vi "_old_Load_SetList_SubVI_Getv2_v4.vi"(0 "Path":path, 1 "error in (no error)":errorcluster) -> (2 "Procedure Name":string="IBS_PICameraTest_29Sep04", 3 "Paramaters":T1 {"Agilent built-in fxns array"."Ring" items=["Agilent", "Rohde & Schwarz"]; "Agilent built-in fxns array"."Agilent phase shift parameter"."FSK pulse length [s]" min=1e-06 max=80000000.0 format="%.3p"; "Agilent built-in fxns array"."Agilent phase shift parameter"."Phase [deg]" min=1e-06 max=80000000.0 format="%.3p"; "Agilent built-in fxns array"."Function selection" items=["Fixed waveform", "Frequency sweep", "Phase shift"]; "Agilent built-in fxns array"."Agilent selection" items=["Raman"]; "Agilent built-in fxns array"."Agilent fixed waveform parameters"."Amplitude [Vpp]" min=0.001 max=20.0 format="%.2f"; "Agilent built-in fxns array"."Agilent fixed waveform parameters"."Waveform Shape" items=["DC"=0, "Sine"=1, "Square"=2, "Triangle"=3, "Ramp"=4, "Pulse"=6, "Noise"=7, "Sinc"=8, "Neg. Ramp"=9, "Exp. Rise"=10, "Exp. Fall"=11, "Cardiac"=12, "Volatile"=13, "User Def. Wfm"=14]; "Agilent built-in fxns array"."Agilent fixed waveform parameters"."Offset [V]" min=-10.0 max=10.0 format="%.2f"; "Agilent built-in fxns array"."Agilent fixed waveform parameters"."Frequency [Hz]" min=0.0001 max=80000000.0 format="%.6p"; "Agilent built-in fxns array"."Agilent sweep parameters"."Sweep Time [s]" min=0.001 max=500.0 format="%.3p"; "Agilent built-in fxns array"."Agilent sweep parameters"."Sweep Spacing (0: Linear up)" items=["Linear up", "Log up", "Linear down", "Log down"]; "Agilent built-in fxns array"."Agilent sweep parameters"."Sweep Mode (0: Off)" items=["Off", "Int", "Ext", "Bus"]; "Agilent built-in fxns array"."Agilent sweep parameters"."Upper Frequency [Hz][1]" min=1e-06 max=80000000.0 format="%.6p"; "Agilent built-in fxns array"."Agilent sweep parameters"."Lower Frequency [Hz][0]" min=1e-06 max=80000000.0 format="%.6p"; "SRS Ramps"."lattice ramp"."c" format="%.2p"; "SRS Ramps"."lattice ramp"."b" format="%.2p"; "SRS Ramps"."lattice ramp"."dt" format="%.2p"; "SRS Ramps"."lattice ramp"."a" format="%.2p"; "Sequencing Info"."Computed Step Size" format="%.2p"; "Sequencing Info"."Sequenced Data" format="%.2p"; "Sequencing Info"."End" format="%.2p"; "Sequencing Info"."Start" format="%.2p"; "Evaporation Params"."RF ramp list"."Frequency [MHz]" format="%.4f"; "Slave AO Ramp List"."Stop Values" format="%.2f"; "Slave AO Ramp List"."Start Values" format="%.2f"; "Slave AO Ramp List"."Ramp time" format="%.3p"; "Master AO Ramp List"."Stop Values" format="%.2f"; "Master AO Ramp List"."Start Values" format="%.2f"; "Master AO Ramp List"."Ramp time" format="%.3p"; "Slave AO Staging List" format="%.2f"; "Master AO Staging List" format="%.2f"; "Slave PB Staging List"."Delay (s)" format="%.3p"; "Master PB Staging List"."Delay (s)" format="%.3p"}, 4 "error out":errorcluster)   [LabVIEW 2013]
uses:
  <vilib>/Utility/file.llb/Read From Spreadsheet File (DBL).vi
panel:
  # "Scan Data"
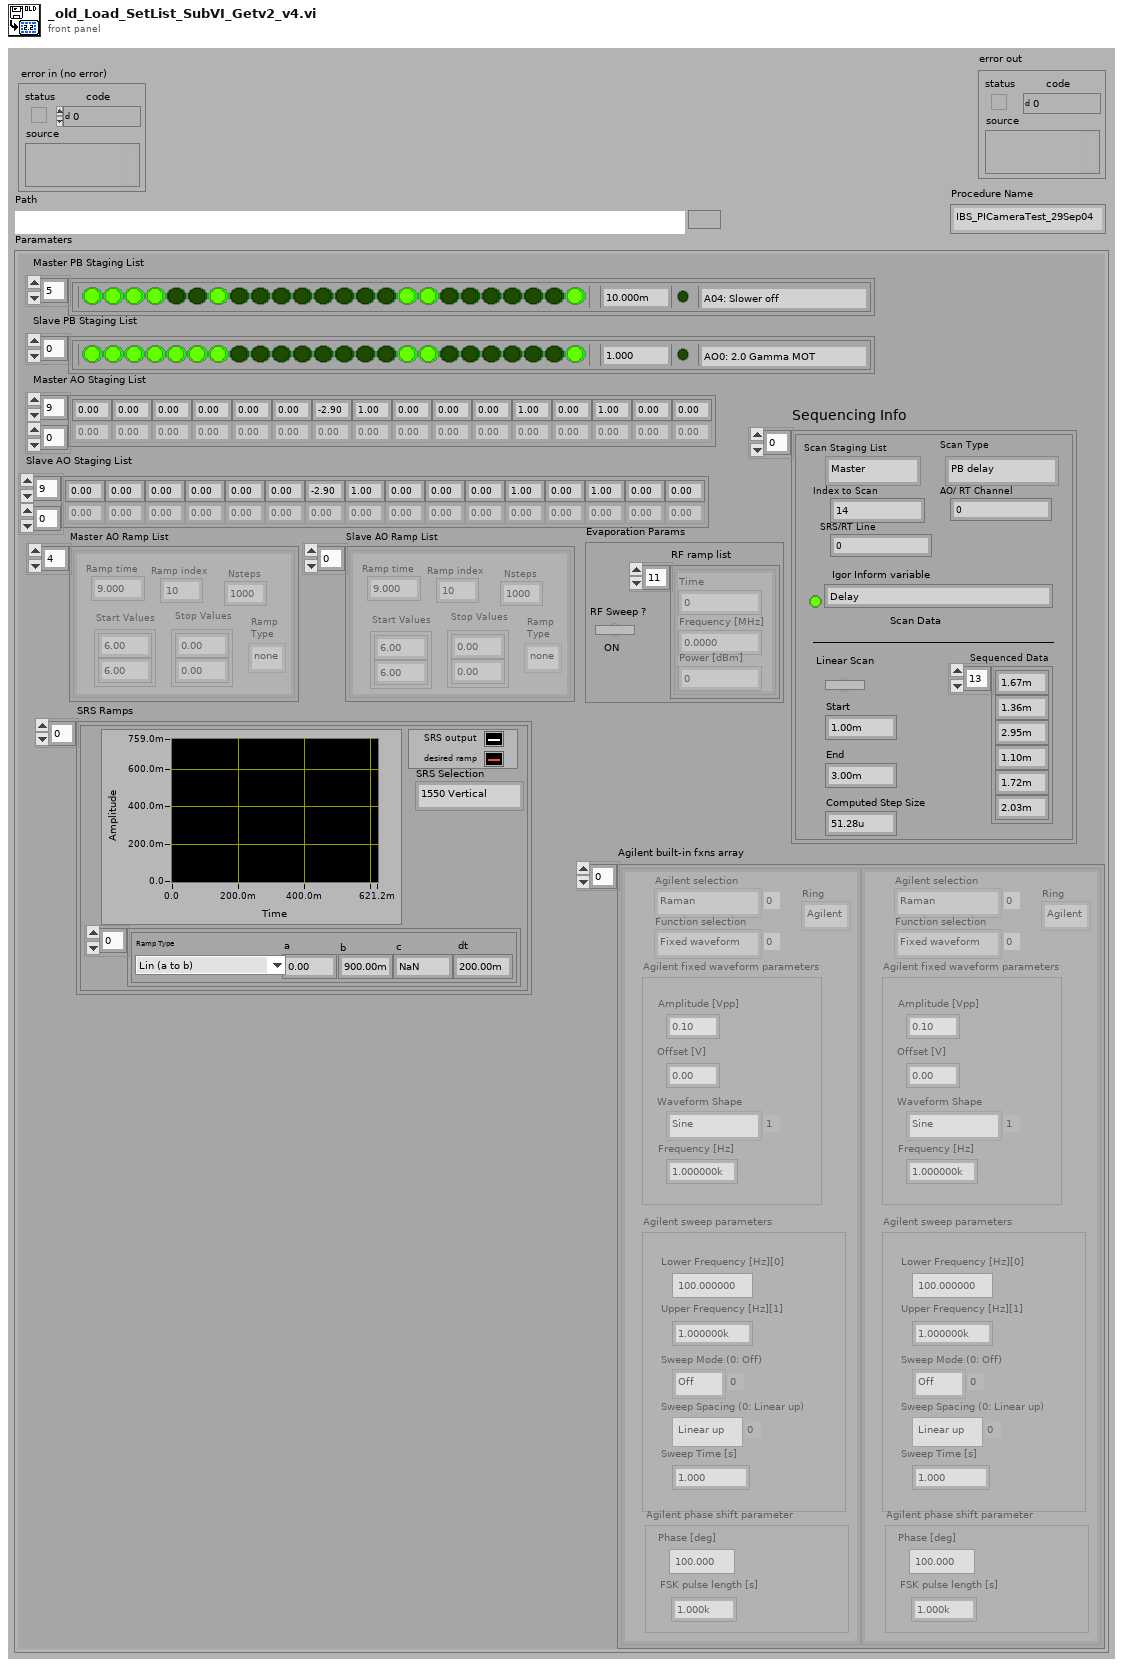
[diagram p1: front panel]
types:
  T1 = cluster{"Master PB Staging List":cluster{"Output Bits":bool[], "Delay (s)":dbl, "String":string, "Halt?":bool}[], "Slave PB Staging List":cluster{"Output Bits":bool[], "Delay (s)":dbl, "String":string, "Halt?":bool}[], "Master AO Staging List":dbl[][], "Slave AO Staging List":dbl[][], "Master AO Ramp List":cluster{"Ramp time":dbl, "Nsteps":u32, "Ramp index":u32, "Start Values":dbl[], "Stop Values":dbl[], "Ramp\nType":enum16{"none", "AO", "AI"}}[], "Slave AO Ramp List":cluster{"Ramp time":dbl, "Nsteps":u32, "Ramp index":u32, "Start Values":dbl[], "Stop Values":dbl[], "Ramp\nType":enum16{"none", "AO", "AI"}}[], "Evaporation Params":cluster{"RF Sweep ?":bool, "RF ramp list":cluster{"Time":dbl, "Frequency [MHz]":dbl, "Power [dBm]":dbl}[]}, "Sequencing Info":cluster{"Start":dbl, "End":dbl, "Sequenced Data":dbl[], "Sequence Data Source":bool, "Scan Staging List":enum16{"Master", "Slave"}, "Index to Scan":i16, "Scan Type":enum16{"PB delay", "AO", "Evap Time", "Evap Amp", "Evap Freq", "Agilent fixed waveform", "Agilent sweep", "Variable Ramp"}, "AO/ RT Channel":i16, "Igor Inform variable":string, "Inform?":bool, "Computed Step Size":dbl, "SRS/RT Line":i16}[], "SRS Ramps":cluster{"lattice ramp":cluster{"a":dbl, "dt":dbl, "Ramp Type":enum16{"Hold=a", "Lin (a to b)", "Exp, (a to b with tau=c)", "Sin=a+b*sin(2*pi*c*t)", "SG a=off, c=f, b=amp", "Blackman (a = amp)", "HGauss (a to b, width c)", "Chirp (a+b*sin(2*pi*f*t)), f from c to d"}, "b":dbl, "c":dbl}[], "Output":cluster{"Time Values":dbl[], dbl[]}[], "SRS Selection":enum16{"1550 Vertical", "Bragg Agilent", "Bragg PTS", "Acc. Intensity"}}[], "Agilent built-in fxns array":cluster{"Agilent sweep parameters":cluster{"Lower Frequency [Hz][0]":dbl, "Upper Frequency [Hz][1]":dbl, "Sweep Mode (0: Off)":u16, "Sweep Spacing (0: Linear up)":u16, "Sweep Time [s]":dbl}, "Agilent fixed waveform parameters":cluster{"Frequency [Hz]":dbl, "Offset [V]":dbl, "Waveform Shape":u16, "Amplitude [Vpp]":dbl}, "Agilent selection":u16, "Function selection":u16, "Agilent phase shift parameter":cluster{"Phase [deg]":dbl, "FSK pulse length [s]":dbl}, "Ring":u16}[]}
  T2 = cluster{"RF Sweep ?":bool, "RF ramp list":cluster{"Time":dbl, "Frequency [MHz]":dbl, "Power [dBm]":dbl}[]}
  T3 = cluster{"Array Constant":bool[], "code":dbl, string, bool}
  T4 = cluster{"Start":dbl, "End":dbl, "Sequenced Data":dbl[], "Sequence Data Source":bool, "Scan Staging List":enum16{"Master", "Slave"}, "Index to Scan":i16, "Scan Type":enum16{"PB delay", "AO", "Evap Time", "Evap Amp", "Evap Freq", "Agilent fixed waveform", "Agilent sweep", "Variable Ramp"}, "AO/ RT Channel":i16, "Igor Inform variable":string, "Inform?":bool, "Computed Step Size":dbl, "SRS/RT Line":i16}
  T5 = cluster{"lattice ramp":cluster{"a":dbl, "dt":dbl, "Ramp Type":enum16{"Hold=a", "Lin (a to b)", "Exp, (a to b with tau=c)", "Sin=a+b*sin(2*pi*c*t)", "SG a=off, c=f, b=amp", "Blackman (a = amp)", "HGauss (a to b, width c)", "Chirp (a+b*sin(2*pi*f*t)), f from c to d"}, "b":dbl, "c":dbl}[], "Output":cluster{"Time Values":dbl[], dbl[]}[], "SRS Selection":enum16{"1550 Vertical", "Bragg Agilent", "Bragg PTS", "Acc. Intensity"}}
  T6 = cluster{"Agilent sweep parameters":cluster{"Lower Frequency [Hz][0]":dbl, "Upper Frequency [Hz][1]":dbl, "Sweep Mode (0: Off)":u16, "Sweep Spacing (0: Linear up)":u16, "Sweep Time [s]":dbl}, "Agilent fixed waveform parameters":cluster{"Frequency [Hz]":dbl, "Offset [V]":dbl, "Waveform Shape":u16, "Amplitude [Vpp]":dbl}, "Agilent selection":u16, "Function selection":u16, "Agilent phase shift parameter":cluster{"Phase [deg]":dbl, "FSK pulse length [s]":dbl}, "Ring":u16}[]
  T7 = cluster{"Ramp time":dbl, "Nsteps":u32, "Ramp index":u32, "Start Values":dbl[], "Stop Values":dbl[], "Ramp\nType":enum16{"none", "AO", "AI"}}
  T8 = cluster{"Ramp time":dbl, "Nsteps":u32, "Ramp index":u32, "Start Values":dbl[], "Stop Values":dbl[], "Ramp\nType":enum16{"none", "AO", "AI"}}[]
  T9 = cluster{"Array Constant":bool[], "code":dbl, string, bool}[]
  T10 = cluster{"Boolean array":bool[], dbl, "output string":string, bool}
  T11 = cluster{"Boolean array":bool[], "code":dbl, "output string":string, bool}[]
  T12 = cluster{"Start":dbl, "End":dbl, "Sequenced Data":dbl[], "Sequence Data Source":bool, "Scan Staging List":enum16{"Master", "Slave"}, "Index to Scan":i16, "Scan Type":enum16{"PB delay", "AO", "Evap Time", "Evap Amp", "Evap Freq", "Agilent fixed waveform", "Agilent sweep", "Variable Ramp"}, "AO/ RT Channel":i16, "Igor Inform variable":string, "Inform?":bool, "Computed Step Size":dbl, "SRS/RT Line":i16}[]
  T13 = cluster{"lattice ramp":cluster{"a":dbl, "dt":dbl, "Ramp Type":enum16{"Hold=a", "Lin (a to b)", "Exp, (a to b with tau=c)", "Sin=a+b*sin(2*pi*c*t)", "SG a=off, c=f, b=amp", "Blackman (a = amp)", "HGauss (a to b, width c)", "Chirp (a+b*sin(2*pi*f*t)), f from c to d"}, "b":dbl, "c":dbl}[], "Output":cluster{"Time Values":dbl[], dbl[]}[], "SRS Selection":enum16{"1550 Vertical", "Bragg Agilent", "Bragg PTS", "Acc. Intensity"}}[]
  T14 = cluster{"Agilent sweep parameters":cluster{"Lower Frequency [Hz][0]":dbl, "Upper Frequency [Hz][1]":dbl, "Sweep Mode (0: Off)":u16, "Sweep Spacing (0: Linear up)":u16, "Sweep Time [s]":dbl}, "Agilent fixed waveform parameters":cluster{"Frequency [Hz]":dbl, "Offset [V]":dbl, "Waveform Shape":u16, "Amplitude [Vpp]":dbl}, "Agilent selection":u16, "Function selection":u16, "Agilent phase shift parameter":cluster{"Phase [deg]":dbl, "FSK pulse length [s]":dbl}, "Ring":u16}
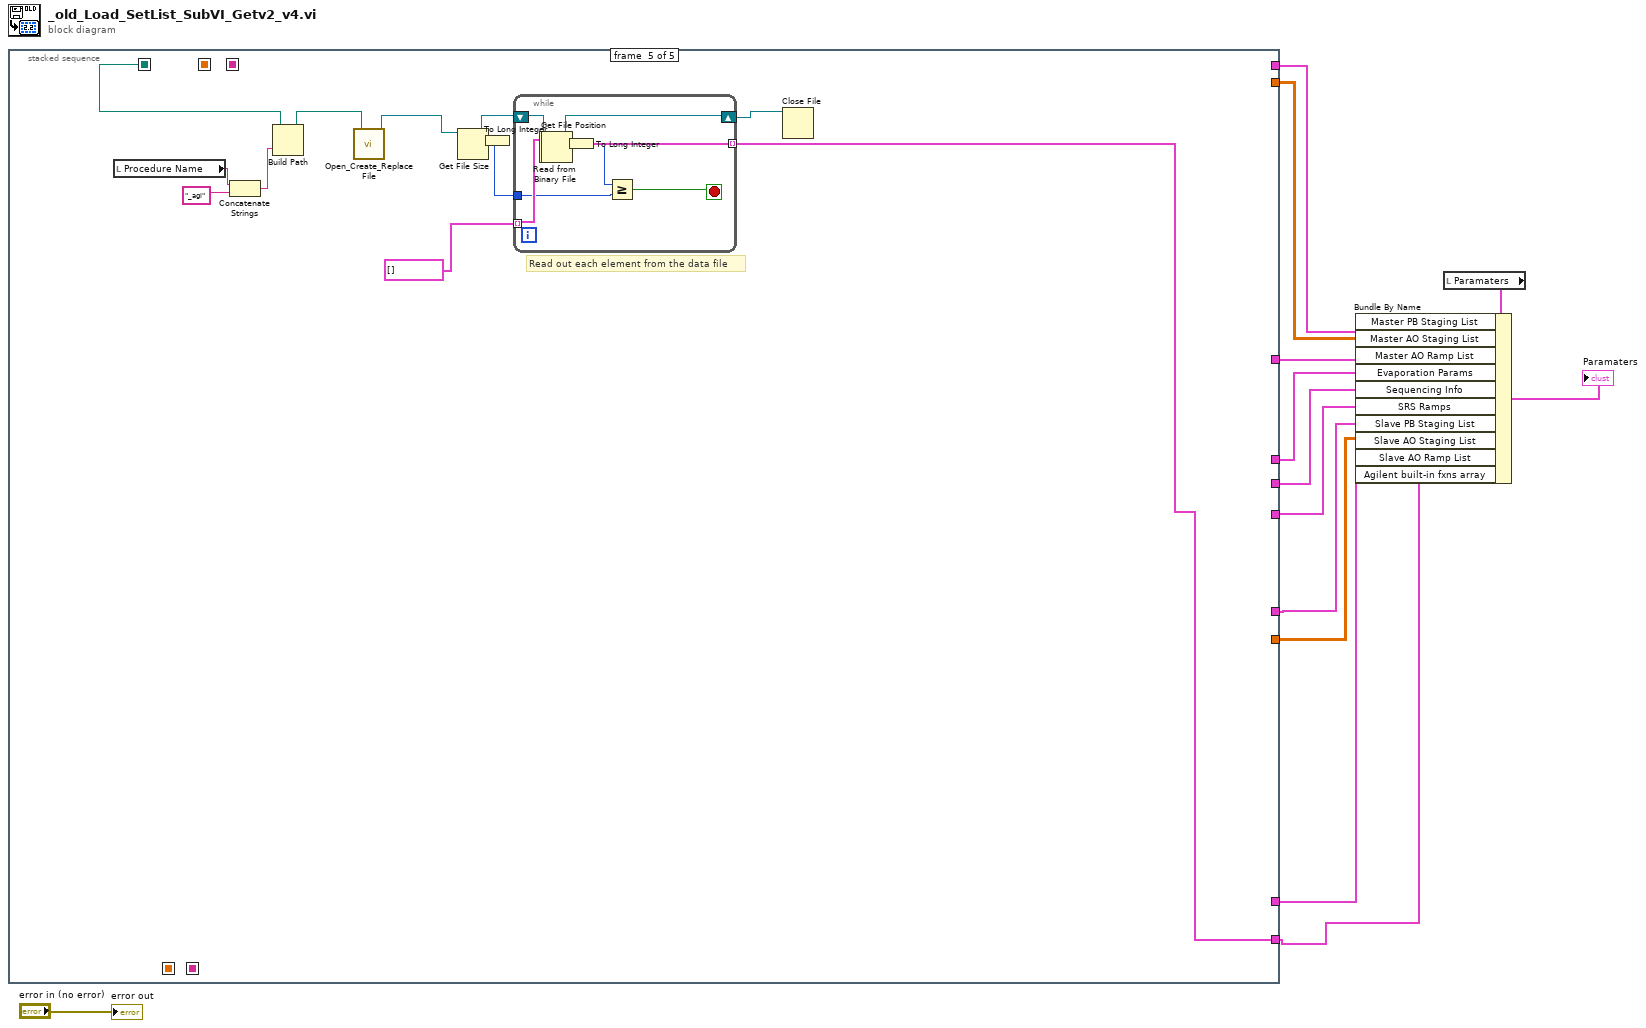
[diagram p0: block diagram]
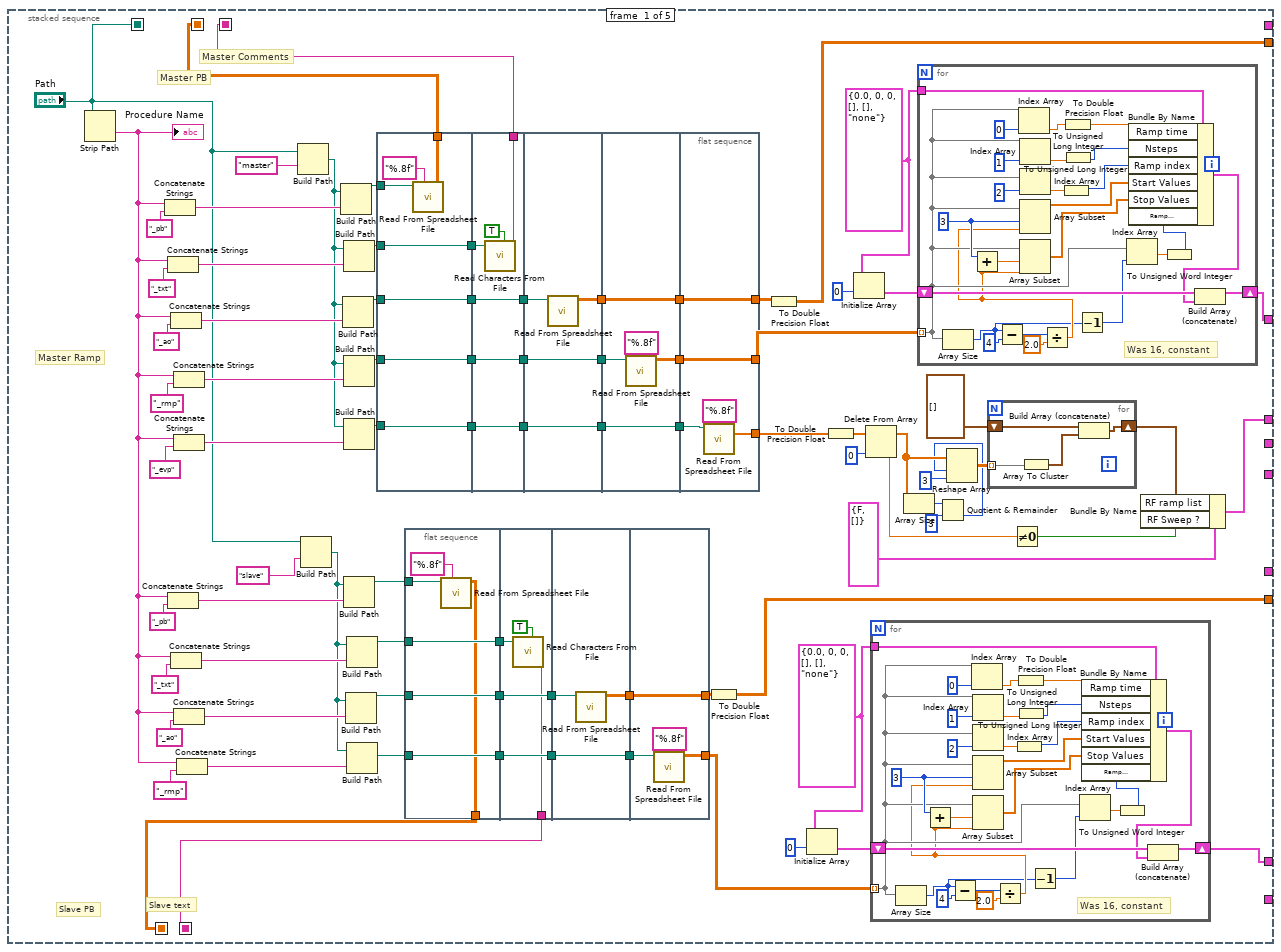
[diagram p2: hidden frame]
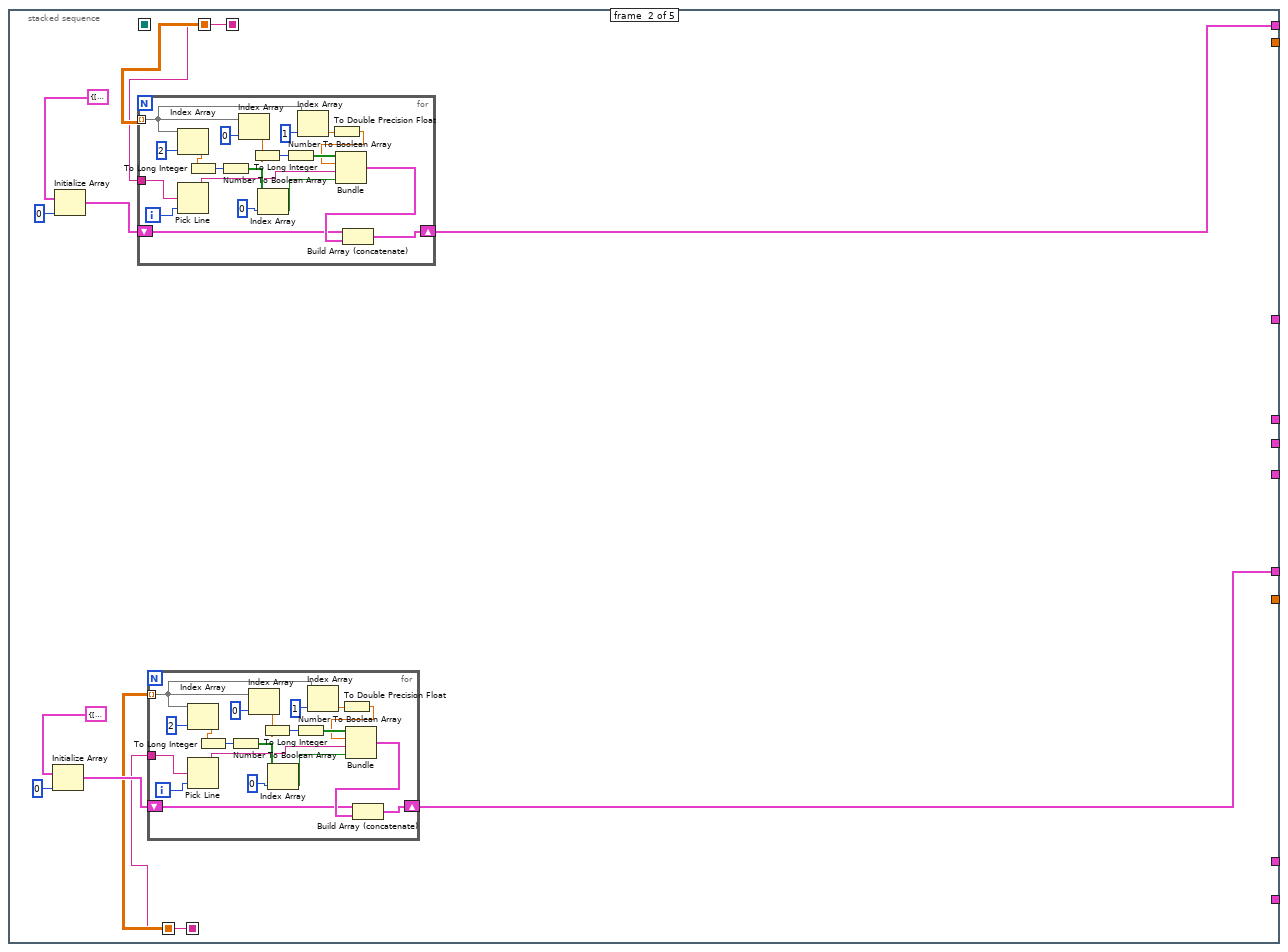
[diagram p3: hidden frame]
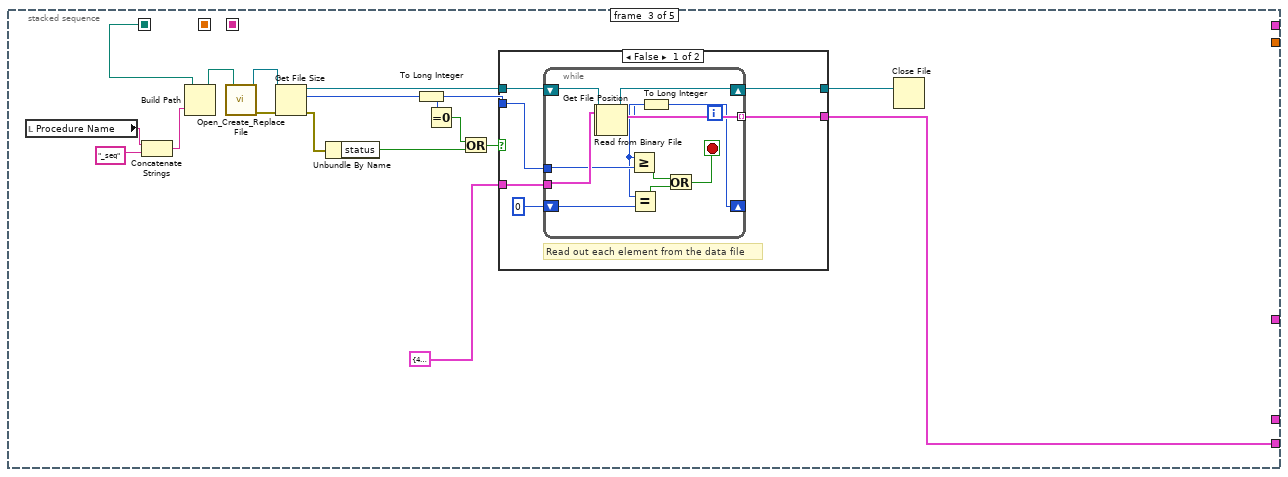
[diagram p4: hidden frame]
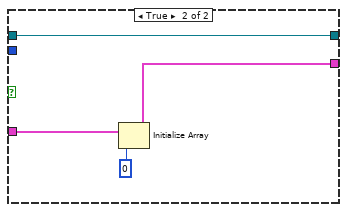
[diagram p5: hidden frame]
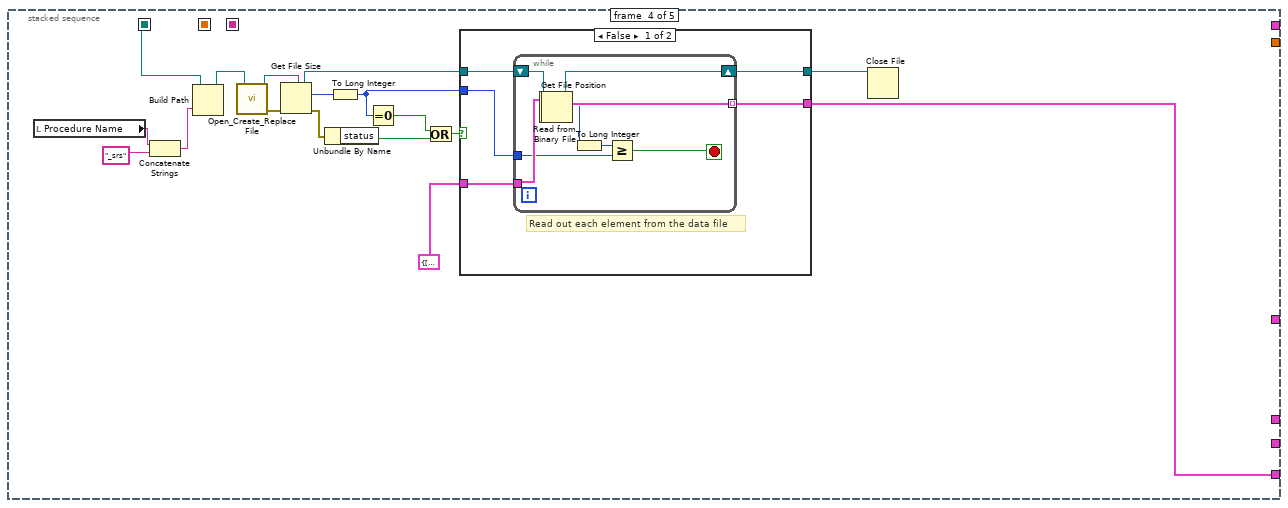
[diagram p6: hidden frame]
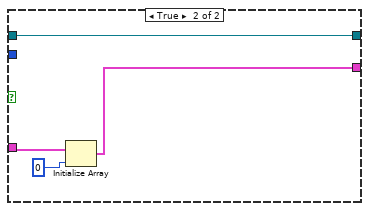
[diagram p7: hidden frame]
diagram:
  n1 = stacked-sequence {
    seq-local: [w72 _ _ _ _] -> [_ w211 _ _ _]
    seq-local: [w56 _ _ _ _] -> [_ w210 _ _ _]
    seq-local: [w30 _ _ _ _] -> [_ w204 _ _ _]
    seq-local: [w31 _ _ _ _] -> [_ w205 _ _ _]
    seq-local: ["Path" _ _ _ _] -> [_ _ w264 w305 w336]
    tunnel: [w26 _ _ _ _] -> w12
    tunnel: [w19 _ _ _ _] -> w11
    tunnel: [w25 _ _ _ _] -> w10
    tunnel: [w24 _ _ _ _] -> w8
    tunnel: [w14 _ _ _ _] -> w7
    tunnel: [_ w202 _ _ _] -> w13
    tunnel: [_ w201 _ _ _] -> w9
    tunnel: [_ _ _ w302 _] -> w6
    tunnel: [_ _ w261 _ _] -> w5
    tunnel: [_ _ _ _ w331] -> w4
    frame #0 {
      w18 = T7 {"Ramp time"=0.0, "Nsteps"=0, "Ramp index"=0, "Start Values"=[], "Stop Values"=[], "Ramp\nType"=enum."none"} ("Ramp Info")
      w23 = T7 {"Ramp time"=0.0, "Nsteps"=0, "Ramp index"=0, "Start Values"=[], "Stop Values"=[], "Ramp\nType"=enum."none"} ("Ramp Info")
      # "Slave text"
      # "Slave PB"
      # "Master Ramp"
      # "Master Comments"
      # "Master PB"
      n2 = Strip Path(path="Path") -> (name=w28:string)  [unwired: 1 out]
      "Procedure Name" <- w28
      n3 = Concatenate Strings(w28, "_pb") -> (w97:string)
      n4 = Concatenate Strings(w28, "_txt") -> (w92:string)
      n5 = Concatenate Strings(w28, "_pb") -> (w85:string)
      n6 = Concatenate Strings(w28, "_ao") -> (w91:string)
      n7 = Concatenate Strings(w28, "_txt") -> (w81:string)
      n8 = Concatenate Strings(w28, "_rmp") -> (w90:string)
      n9 = Concatenate Strings(w28, "_evp") -> (w88:string)
      n10 = Concatenate Strings(w28, "_ao") -> (w80:string)
      n11 = Concatenate Strings(w28, "_rmp") -> (w79:string)
      n12 = Build Path(base path="Path", name or relative path="master") -> (appended path=w89:path)
      n13 = Build Path(base path="Path", name or relative path="slave") -> (appended path=w78:path)
      n14 = Build Path(base path=w89, name or relative path=w97) -> (appended path=w76:path)
      n15 = Build Path(base path=w89, name or relative path=w91) -> (appended path=w74:path)
      n16 = Build Path(base path=w89, name or relative path=w92) -> (appended path=w75:path)
      n17 = Build Path(base path=w89, name or relative path=w90) -> (appended path=w77:path)
      n18 = Build Path(base path=w89, name or relative path=w88) -> (appended path=w73:path)
      n19 = Build Path(base path=w78, name or relative path=w85) -> (appended path=w35:path)
      n20 = Build Path(base path=w78, name or relative path=w80) -> (appended path=w33:path)
      n21 = Build Path(base path=w78, name or relative path=w81) -> (appended path=w34:path)
      n22 = Build Path(base path=w78, name or relative path=w79) -> (appended path=w32:path)
      n23 = flat-sequence {
        tunnel: w77 -> [w171]
        tunnel: w76 -> [w175]
        tunnel: w75 -> [w173]
        tunnel: w74 -> [w172]
        tunnel: w73 -> [w170]
        tunnel: [w174] -> w72
        tunnel: [w173] -> w55
        tunnel: [w172] -> w53
        tunnel: [w171] -> w51
        tunnel: [w170] -> w46
        tunnel: [w180] -> w56
        tunnel: w55 -> [w181]
        tunnel: [w179] -> w54
        tunnel: w53 -> [w179]
        tunnel: w51 -> [w178]
        tunnel: [w178] -> w50
        tunnel: w46 -> [w177]
        tunnel: [w177] -> w45
        tunnel: w54 -> [w185]
        tunnel: [w186] -> w52
        tunnel: w50 -> [w184]
        tunnel: [w184] -> w49
        tunnel: w45 -> [w183]
        tunnel: [w183] -> w44
        tunnel: w52 -> [w191]
        tunnel: w49 -> [w189]
        tunnel: [w191] -> w48
        tunnel: [w188] -> w47
        tunnel: w44 -> [w187]
        tunnel: [w187] -> w43
        tunnel: [w195] -> w20
        tunnel: [w192] -> w70
        tunnel: [w196] -> w71
        tunnel: w48 -> [w196]
        tunnel: w47 -> [w195]
        tunnel: w43 -> [w193]
        frame #0 {
          n24 = call-poly <vilib>:"Read From Spreadsheet File.vi"("format (%.3f)"="%.8f", "file path (dialog if empty)"=w175) -> ("all rows"=w174:dbl[][])  [unwired: 2 in, 7 out]
        }
        frame #1 {
          n25 = call <vilib>:"Read Characters From File.vi"("file path (dialog if empty)"=w181, "convert eol? (no:F)"=TRUE) -> ("character string"=w180:string)  [unwired: 1 in, 6 out]
        }
        frame #2 {
          n26 = call-poly <vilib>:"Read From Spreadsheet File.vi"("file path (dialog if empty)"=w185) -> ("all rows"=w186:dbl[][])  [unwired: 3 in, 7 out]
        }
        frame #3 {
          n27 = call-poly <vilib>:"Read From Spreadsheet File.vi"("format (%.3f)"="%.8f", "file path (dialog if empty)"=w189) -> ("all rows"=w188:dbl[][])  [unwired: 2 in, 7 out]
        }
        frame #4 {
          n28 = call-poly <vilib>:"Read From Spreadsheet File.vi"("format (%.3f)"="%.8f", "file path (dialog if empty)"=w193) -> ("first row"=w192:dbl[])  [unwired: 2 in, 7 out]
        }
      }
      n29 = flat-sequence {
        tunnel: w32 -> [w153]
        tunnel: w35 -> [w156]
        tunnel: w34 -> [w155]
        tunnel: w33 -> [w154]
        tunnel: [w155] -> w42
        tunnel: [w154] -> w41
        tunnel: [w153] -> w40
        tunnel: [w152] -> w31
        tunnel: w42 -> [w161]
        tunnel: [w160] -> w39
        tunnel: w41 -> [w160]
        tunnel: w40 -> [w159]
        tunnel: [w159] -> w38
        tunnel: [w158] -> w30
        tunnel: w39 -> [w164]
        tunnel: [w165] -> w37
        tunnel: w38 -> [w163]
        tunnel: [w163] -> w36
        tunnel: [w166] -> w15
        tunnel: [w169] -> w29
        tunnel: w37 -> [w169]
        tunnel: w36 -> [w167]
        frame #0 {
          n30 = call-poly <vilib>:"Read From Spreadsheet File.vi"("format (%.3f)"="%.8f", "file path (dialog if empty)"=w156) -> ("all rows"=w152:dbl[][])  [unwired: 2 in, 7 out]
        }
        frame #1 {
          n31 = call <vilib>:"Read Characters From File.vi"("file path (dialog if empty)"=w161, "convert eol? (no:F)"=TRUE) -> ("character string"=w158:string)  [unwired: 1 in, 6 out]
        }
        frame #2 {
          n32 = call-poly <vilib>:"Read From Spreadsheet File.vi"("file path (dialog if empty)"=w164) -> ("all rows"=w165:dbl[][])  [unwired: 3 in, 7 out]
        }
        frame #3 {
          n33 = call-poly <vilib>:"Read From Spreadsheet File.vi"("format (%.3f)"="%.8f", "file path (dialog if empty)"=w167) -> ("all rows"=w166:dbl[][])  [unwired: 2 in, 7 out]
        }
      }
      n34 = To Double Precision Float(number=w29) -> (double precision float=w24:dbl[][])
      n35 = To Double Precision Float(number=w71) -> (double precision float=w26:dbl[][])
      n36 = Initialize Array(w18, 0) -> (w17:T8)
      n37 = To Double Precision Float(number=w70) -> (double precision float=w57:dbl[])
      n38 = Initialize Array(w23, 0) -> (w22:T8)
      n39 = Delete From Array(array=w57, index=0) -> (deleted portion=w65:dbl, array with subset deleted=w62:dbl[])  [unwired: 1 in]
      n40 = for {
        tunnel: w15 -> [w106] mode=indexing
        shift-right: [w118] -> w14
        shift-left: w17 -> [w117]
        tunnel: w18 -> [w109]
        w108 = 3
        # "Was 16, constant"
        n41 = Array Size(array=w106) -> (size(s)=w100:i32)
        n42 = Subtract(x=w100, y=4) -> (x-y=w103:i32)
        n43 = Index Array(array=w106, index=0) -> (element=w122:dbl)
        n44 = Index Array(array=w106, index=1) -> (element=w121:dbl)
        n45 = Index Array(array=w106, index=2) -> (element=w120:dbl)
        n46 = Divide(x=w103, y=2.0) -> (x/y=w102:dbl)
        n47 = Add(x=w108, y=w102) -> (x+y=w107:dbl)
        n48 = Array Subset(array=w106, index=w108, length=w102) -> (w113:dbl[])
        n49 = Array Subset(array=w106, index=w107, length=w102) -> (w112:dbl[])
        n50 = To Unsigned Long Integer(number=w120) -> (unsigned 32bit integer=w114:u32)
        n51 = To Double Precision Float(number=w122) -> (double precision float=w116:dbl)
        n52 = To Unsigned Long Integer(number=w121) -> (unsigned 32bit integer=w115:u32)
        n53 = Decrement(x=w100) -> (x-1=w101:i32)
        n54 = Index Array(array=w106, index=w101) -> (element=w119:dbl)
        n55 = To Unsigned Word Integer(number=w119) -> (unsigned 16bit integer=w111:u16)
        n56 = Bundle By Name(cluster=w109, "Ramp time"=w116, "Nsteps"=w115, "Ramp index"=w114, "Start Values"=w113, "Stop Values"=w112, "Ramp\nType"=w111) -> (w110:T7)
        n57 = Build Array (concatenate)(w117, w110) -> (w118:T8)
      }
      n58 = Array Size(array=w62) -> (size(s)=w61:i32)
      n59 = for {
        tunnel: w20 -> [w132] mode=indexing
        shift-right: [w144] -> w19
        shift-left: w22 -> [w143]
        tunnel: w23 -> [w135]
        w134 = 3
        # "Was 16, constant"
        n60 = Array Size(array=w132) -> (size(s)=w126:i32)
        n61 = Subtract(x=w126, y=4) -> (x-y=w129:i32)
        n62 = Index Array(array=w132, index=0) -> (element=w148:dbl)
        n63 = Index Array(array=w132, index=1) -> (element=w147:dbl)
        n64 = Index Array(array=w132, index=2) -> (element=w146:dbl)
        n65 = Divide(x=w129, y=2.0) -> (x/y=w128:dbl)
        n66 = Add(x=w134, y=w128) -> (x+y=w133:dbl)
        n67 = Array Subset(array=w132, index=w134, length=w128) -> (w139:dbl[])
        n68 = Array Subset(array=w132, index=w133, length=w128) -> (w138:dbl[])
        n69 = To Unsigned Long Integer(number=w146) -> (unsigned 32bit integer=w140:u32)
        n70 = To Double Precision Float(number=w148) -> (double precision float=w142:dbl)
        n71 = To Unsigned Long Integer(number=w147) -> (unsigned 32bit integer=w141:u32)
        n72 = Decrement(x=w126) -> (x-1=w127:i32)
        n73 = Index Array(array=w132, index=w127) -> (element=w145:dbl)
        n74 = To Unsigned Word Integer(number=w145) -> (unsigned 16bit integer=w137:u16)
        n75 = Bundle By Name(cluster=w135, "Ramp time"=w142, "Nsteps"=w141, "Ramp index"=w140, "Start Values"=w139, "Stop Values"=w138, "Ramp\nType"=w137) -> (w136:T7)
        n76 = Build Array (concatenate)(w143, w136) -> (w144:T8)
      }
      n77 = Quotient & Remainder(x=w61, y=3) -> (floor(x/y)=w58:i32)  [unwired: 1 out]
      n78 = Reshape Array(w62, w58, 3) -> (w63:dbl[][])
      n79 = for {
        tunnel: w63 -> [w198] mode=indexing
        shift-right: [w200] -> w67
        shift-left: cluster{dbl, dbl, dbl}[] [] -> [w199]
        n80 = Array To Cluster(array=w198) -> (cluster=w197:cluster{"[0]":dbl, "[1]":dbl, "[2]":dbl})
        n81 = Build Array (concatenate)(w199, w197) -> (w200:cluster{"[0]":dbl, "[1]":dbl, "[2]":dbl}[])
      }
      n82 = Not Equal To 0?(x=w65) -> (x != 0?=w64:bool)
      n83 = Bundle By Name(cluster=T2 {"RF Sweep ?"=FALSE, "RF ramp list"=[]} ("Evaporation Params"), "RF ramp list"=w67, "RF Sweep ?"=w64) -> (w25:T2)
    }
    frame #1 {
      n84 = Initialize Array(T3 {"Array Constant"=[], "code"=0.0, "", TRUE}, 0) -> (w207:T9)
      n85 = Initialize Array(T3 {"Array Constant"=[], "code"=0.0, "", TRUE}, 0) -> (w203:T9)
      n86 = for {
        tunnel: w211 -> [w242] mode=indexing
        tunnel: w210 -> [w252]
        shift-right: [w234] -> w202
        shift-left: w203 -> [w233]
        i -> [w246]
        n87 = Index Array(array=w242, index=2 ("Index")) -> (element=w241:dbl)
        n88 = Pick Line(multi-line string=w252, line index=w246) -> (output string=w236:string)  [unwired: 1 out]
        n89 = To Long Integer(number=w241) -> (32bit integer=w240:i32)
        n90 = Number To Boolean Array(number=w240) -> (Boolean array=w238:bool[])
        n91 = Index Array(array=w242, index=0) -> (element=w250:dbl)
        n92 = To Long Integer(number=w250) -> (32bit integer=w249:i32)
        n93 = Index Array(array=w238, index=0) -> (element=w237:bool)
        n94 = Number To Boolean Array(number=w249) -> (Boolean array=w251:bool[])
        n95 = Index Array(array=w242, index=1) -> (element=w248:dbl)
        n96 = To Double Precision Float(number=w248) -> (double precision float=w247:dbl)
        n97 = Bundle("Boolean array"=w251, w247, "output string"=w236, w237) -> (w235:T10)  [unwired: 1 out]
        n98 = Build Array (concatenate)(w233, w235) -> (w234:T11)
      }
      n99 = for {
        tunnel: w205 -> [w222] mode=indexing
        tunnel: w204 -> [w232]
        shift-right: [w214] -> w201
        shift-left: w207 -> [w213]
        i -> [w226]
        n100 = Index Array(array=w222, index=2 ("Index")) -> (element=w221:dbl)
        n101 = Pick Line(multi-line string=w232, line index=w226) -> (output string=w216:string)  [unwired: 1 out]
        n102 = To Long Integer(number=w221) -> (32bit integer=w220:i32)
        n103 = Number To Boolean Array(number=w220) -> (Boolean array=w218:bool[])
        n104 = Index Array(array=w222, index=0) -> (element=w230:dbl)
        n105 = To Long Integer(number=w230) -> (32bit integer=w229:i32)
        n106 = Index Array(array=w218, index=0) -> (element=w217:bool)
        n107 = Number To Boolean Array(number=w229) -> (Boolean array=w231:bool[])
        n108 = Index Array(array=w222, index=1) -> (element=w228:dbl)
        n109 = To Double Precision Float(number=w228) -> (double precision float=w227:dbl)
        n110 = Bundle("Boolean array"=w231, w227, "output string"=w216, w217) -> (w215:T10)  [unwired: 1 out]
        n111 = Build Array (concatenate)(w213, w215) -> (w214:T11)
      }
    }
    frame #2 {
      n112 = local read "Procedure Name"() -> (w268:string)
      n113 = Concatenate Strings(w268, "_seq") -> (w265:string)
      n114 = Build Path(base path=w264, name or relative path=w265) -> (appended path=w269:path)
      n115 = call <vilib>:"Open_Create_Replace File.vi"("file path"=w269) -> ("error out"=w254:errorcluster, "refnum"=w263:refnum<file>)  [unwired: 5 in, 4 out]
      n116 = Get File Size(file=w263, error in=w254) -> (refnum out=w262:refnum<file>, size (in bytes)=w259:i64, 0:w253:errorcluster)
      n117 = Unbundle By Name(w253) -> ("status"=w255:bool)
      n118 = To Long Integer(number=w259) -> (32bit integer=w260:i32)
      n119 = Equal To 0?(x=w260) -> (x = 0?=w256:bool)
      n120 = Or(x=w256, y=w255) -> (x .or. y?=w257:bool)
      n121 = case shown="False" w257 {
        tunnel: [w275 w292] -> w267
        tunnel: T4 {"Start"=4.0, "End"=-20.0, "Sequenced Data"=[2.0, -18.0, -2.0, -4.0, -13.0, -1.0, -20.0, -10.0, -11.0, -7.0, 0.0, 3.0, -15.0, 4.0, -12.0, 1.0, -6.0, -9.0, -14.0, -16.0, -3.0, -17.0, -8.0, -19.0, -5.0], "Sequence Data Source"=FALSE, "Scan Staging List"=enum."Master", "Index to Scan"=6, "Scan Type"=enum."Evap Amp", "AO/ RT Channel"=9, "Igor Inform variable"="Delay", "Inform?"=TRUE, "Computed Step Size"=-1.0, "SRS/RT Line"=9} ("Sequencing Info") -> [w274 w290]
        tunnel: w262 -> [w273 w292]
        tunnel: [w272 w291] -> w261
        tunnel: w260 -> [w271 _]
        frame False {
          # "Read out each element from the data file"
          n122 = while {
            tunnel: [w286] -> w272 mode=indexing
            tunnel: w274 -> [w285]
            shift-right: [w287] -> w275
            shift-left: w273 -> [w288]
            tunnel: w271 -> [w284]
            shift-right: [w283] -> _
            shift-left: 0 -> [w282]
            stop <- w279 stop-if-true
            n123 = Read from Binary File(5:w285, 11:w288) -> (0:w277:errorcluster, 2:w286:T4, 3:w278:refnum<file>)  [unwired: 1 in, 4 out]
            n124 = Get File Position(4:w277, 7:w278) -> (2:w276:i64, 3:w287:refnum<file>)  [unwired: 1 out]
            n125 = To Long Integer(number=w276) -> (32bit integer=w283:i32)
            n126 = Greater Or Equal?(x=w283, y=w284) -> (x >= y?=w280:bool)
            n127 = Equal?(x=w283, y=w282) -> (x = y?=w281:bool)
            n128 = Or(x=w280, y=w281) -> (x .or. y?=w279:bool)
          }
        }
        frame True {
          n129 = Initialize Array(w290, 0) -> (w291:T12)
        }
      }
      n130 = Close File(refnum=w267) -> ()  [unwired: 1 in, 2 out]
    }
    frame #3 {
      n131 = local read "Procedure Name"() -> (w308:string)
      n132 = Concatenate Strings(w308, "_srs") -> (w306:string)
      n133 = Build Path(base path=w305, name or relative path=w306) -> (appended path=w309:path)
      n134 = call <vilib>:"Open_Create_Replace File.vi"("file path"=w309) -> ("error out"=w293:errorcluster, "refnum"=w301:refnum<file>)  [unwired: 5 in, 4 out]
      n135 = Get File Size(file=w301, error in=w293) -> (refnum out=w304:refnum<file>, size (in bytes)=w299:i64, 0:w294:errorcluster)
      n136 = Unbundle By Name(w294) -> ("status"=w295:bool)
      n137 = To Long Integer(number=w299) -> (32bit integer=w298:i32)
      n138 = Equal To 0?(x=w298) -> (x = 0?=w296:bool)
      n139 = Or(x=w296, y=w295) -> (x .or. y?=w297:bool)
      n140 = case shown="False" w297 {
        tunnel: w304 -> [w314 w328]
        tunnel: [w313 w328] -> w303
        tunnel: [w312 w325] -> w302
        tunnel: T5 {"lattice ramp"=[{"a"=0.0, "dt"=0.00101, "Ramp Type"=enum."Hold=a", "b"=nan, "c"=nan}, {"a"=0.42, "dt"=2e-05, "Ramp Type"=enum."Hold=a", "b"=0.42, "c"=0.08}, {"a"=0.0, "dt"=5e-06, "Ramp Type"=enum."Hold=a", "b"=nan, "c"=nan}, {"a"=0.0, "dt"=1e-05, "Ramp Type"=enum."Hold=a", "b"=0.0, "c"=-0.0001}, {"a"=0.0, "dt"=0.0001, "Ramp Type"=enum."Hold=a", "b"=nan, "c"=nan}, {"a"=2.0, "dt"=0.0001, "Ramp Type"=enum."Hold=a", "b"=nan, "c"=nan}], "Output"=[{"Time Values"=[0.0, 1e-07, 0.0005049999999999999, 0.0010099, 0.00101, 0.00102, 0.00103, 0.0010301000000000002, 0.0010325000000000002, 0.0010349, 0.0010350000000000001, 0.0010400000000000001, 0.0010450000000000001, 0.0010451000000000002, 0.0010950000000000003, 0.0011449000000000001, 0.0011450000000000002, 0.001195, 0.0012450000000000002], [2.0, 0.0, 0.0, 0.0, 0.42, 0.42, 0.42, 0.0, 0.0, 0.0, 0.0, 0.0, 0.0, 0.0, 0.0, 0.0, 2.0, 2.0, 2.0]}, {"Time Values"=[0.0, 1e-07, 0.0005049999999999999, 0.0010099, 0.00101, 0.00102, 0.00103, 0.0010301000000000002, 0.0010325000000000002, 0.0010349, 0.0010350000000000001, 0.0010400000000000001, 0.0010450000000000001, 0.0010451000000000002, 0.0010950000000000003, 0.0011449000000000001, 0.0011450000000000002, 0.001195, 0.0012450000000000002], [2.0, 0.0, 0.0, 0.0, 0.42, 0.42, 0.42, 0.0, 0.0, 0.0, 0.0, 0.0, 0.0, 0.0, 0.0, 0.0, 2.0, 2.0, 2.0]}], "SRS Selection"=enum."Bragg Agilent"} ("Ramp") -> [w311 w327]
        tunnel: w298 -> [w310 _]
        frame False {
          # "Read out each element from the data file"
          n141 = while {
            tunnel: [w322] -> w312 mode=indexing
            tunnel: w311 -> [w321]
            shift-right: [w323] -> w313
            shift-left: w314 -> [w324]
            tunnel: w310 -> [w320]
            stop <- w318 stop-if-true
            n142 = Read from Binary File(5:w321, 11:w324) -> (0:w316:errorcluster, 2:w322:T5, 3:w317:refnum<file>)  [unwired: 1 in, 4 out]
            n143 = Get File Position(4:w316, 7:w317) -> (2:w315:i64, 3:w323:refnum<file>)  [unwired: 1 out]
            n144 = To Long Integer(number=w315) -> (32bit integer=w319:i32)
            n145 = Greater Or Equal?(x=w319, y=w320) -> (x >= y?=w318:bool)
          }
        }
        frame True {
          n146 = Initialize Array(w327, 0) -> (w325:T13)
        }
      }
      n147 = Close File(refnum=w303) -> ()  [unwired: 1 in, 2 out]
    }
    frame #4 {
      # "Read out each element from the data file"
      n148 = local read "Procedure Name"() -> (w339:string)
      n149 = Concatenate Strings(w339, "_agi") -> (w337:string)
      n150 = Build Path(base path=w336, name or relative path=w337) -> (appended path=w340:path)
      n151 = call <vilib>:"Open_Create_Replace File.vi"("file path"=w340) -> ("refnum"=w332:refnum<file>)  [unwired: 5 in, 5 out]
      n152 = Get File Size(file=w332) -> (refnum out=w335:refnum<file>, size (in bytes)=w330:i64)  [unwired: 1 in, 1 out]
      n153 = To Long Integer(number=w330) -> (32bit integer=w334:i32)
      n154 = while {
        tunnel: [w348] -> w331 mode=indexing
        tunnel: T6 [] ("Agilent built-in fxns array") -> [w347] mode=indexing
        shift-right: [w349] -> w333
        shift-left: w335 -> [w350]
        tunnel: w334 -> [w346]
        stop <- w344 stop-if-true
        n155 = Read from Binary File(5:w347, 11:w350) -> (0:w342:errorcluster, 2:w348:T14, 3:w343:refnum<file>)  [unwired: 1 in, 4 out]
        n156 = Get File Position(4:w342, 7:w343) -> (2:w341:i64, 3:w349:refnum<file>)  [unwired: 1 out]
        n157 = To Long Integer(number=w341) -> (32bit integer=w345:i32)
        n158 = Greater Or Equal?(x=w345, y=w346) -> (x >= y?=w344:bool)
      }
      n159 = Close File(refnum=w333) -> ()  [unwired: 1 in, 2 out]
    }
  }
  n160 = local read "Paramaters"() -> (w2:T1)
  n161 = Bundle By Name(cluster=w2, "Master PB Staging List"=w13, "Master AO Staging List"=w12, "Master AO Ramp List"=w11, "Evaporation Params"=w10, "Sequencing Info"=w5, "SRS Ramps"=w6, "Slave PB Staging List"=w9, "Slave AO Staging List"=w8, "Slave AO Ramp List"=w7, "Agilent built-in fxns array"=w4) -> (→"Paramaters":T1)
  "error out" <- "error in (no error)"
